vi "Read Peak Data from File.vi"(8 "error in (no error)":errorcluster, 11 "Data File":path) -> (0 "error out":errorcluster, 3 "Peaks":string[][](array[string]))   [LabVIEW 2020, in "Waters Patrol UPLC Report Parser.lvlib" / "Instrument Manager.lvlib"]
uses:
  Instrument Manager.lvlib
  <vilib>/Utility/file.llb/Read Delimited Spreadsheet (string).vi
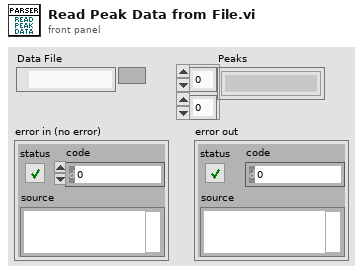
[diagram p1: front panel]
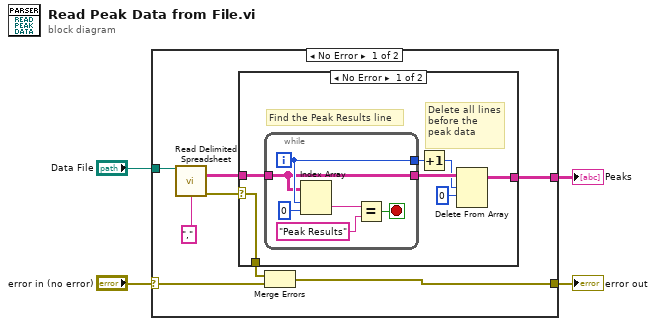
[diagram p0: block diagram]
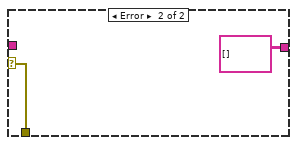
[diagram p2: hidden frame]
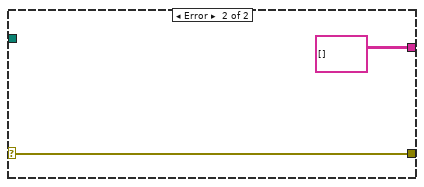
[diagram p3: hidden frame]
diagram:
  n1 = case shown="No Error" "error in (no error)" {
    selector: "error in (no error)" -> [w9 w29]
    tunnel: [w12 string[][] [] ("all rows")] -> w4
    tunnel: "Data File" -> [w10 _]
    tunnel: [w6 w29] -> w1
    frame No Error {
      n2 = call-poly <vilib>:"Read Delimited Spreadsheet.vi"("file path (dialog if empty)"=w10, "delimiter (\\t)"="," ("delimiter (\\t)")) -> ("all rows"=w11:string[][], "error out"=w7:errorcluster)  [unwired: 8 in, 4 out]
      n3 = case shown="No Error" w7 {
        selector: w7 -> [w13 w27]
        tunnel: [w19 string[][] [] ("all rows")] -> w12
        tunnel: w11 -> [w15 _]
        tunnel: [w13 w27] -> w5
        frame No Error {
          # "Find the Peak Results line"
          # "Delete all lines\nbefore the\npeak data"
          n4 = while {
            tunnel: w15 -> [w20]
            tunnel: [w21] -> w17
            tunnel: [w20] -> w16
            i -> [w21]
            stop <- w22 stop-if-true
            n5 = Index Array(array=w20, index (row)=w21, index (col)=0 ("index (row)")) -> (element=w24:string)
            n6 = Equal?(x=w24, y="Peak Results") -> (x = y?=w22:bool)
          }
          n7 = Increment(x=w17) -> (x+1=w14:i32)
          n8 = Delete From Array(array=w16, length=w14, index (row)=0) -> (array with subset deleted=w19:string[][])  [unwired: 1 in, 1 out]
        }
        frame Error {
        }
      }
      n9 = Merge Errors(w5, w9) -> (w6:errorcluster)
    }
    frame Error {
    }
  }
  "Peaks" <- w4
  "error out" <- w1
